vi "Standard Event Status Enable.vi"(0 "VISA resource name":refnum<visa-resource-name>, 5 "Standard Event Status Enable":T1, 11 "error in (no error)":errorcluster) -> (4 "VISA resource name out":refnum<visa-resource-name>, 15 "error out":errorcluster)   [LabVIEW 2014, in "Associated Power Technologies 8500 Series.lvlib"]
doc: "Enables the events for which the status is to be monitored in the instrument.\n\nThe Standard Event Register consists of the following 8 bits.\nBit 0: Operation Complete\nBit 1: not used\nBit 2: Query Error \nBit 3: Device Error\nBit 4: Message Available\nBit 5: Command Error \nBit 6: not used\nBit 7: Power On\n\nExample:\nIf the User gives 0|dec (whose binary equivalent is 00000000|bin) to this VI, no event status will be enabled.\n\nIf 255|dec (11111111|bin) is given, all the events (Operation Complete, User Defined, Query Error, Device Error, Message Available, Command Error,User Defined, Power On) will be enabled.\n\n<B>Default</B>: 32|dec=00100000|bin"
uses:
  <instrlib>/Associated Power Technologies 8500 Series/Associated Power Technologies 8500 Series.lvlib
panel:
  # "Bit 0: Operation Complete\nBit 1:  not used\nBit 2:  Query Error\t\nBit 3:  Device Error\nBit 4:\t\tMessage Available\nBit 5:  Command Error\t\nBit 6:  not used\nBit 7:  Power On"
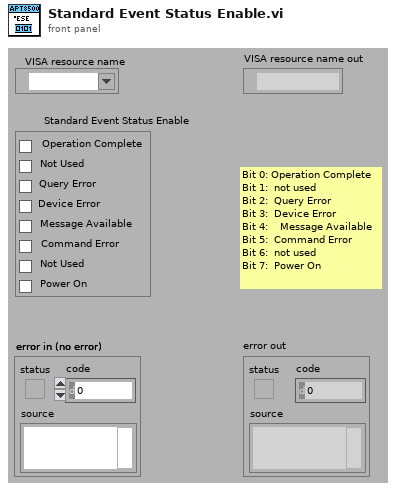
[diagram p1: front panel]
types:
  T1 = cluster{"Operation Complete":bool, "Not Used":bool, "Query Error":bool, "Device Error":bool, "Message Available":bool, "Command Error":bool, "Not Used":bool, "Power On":bool}
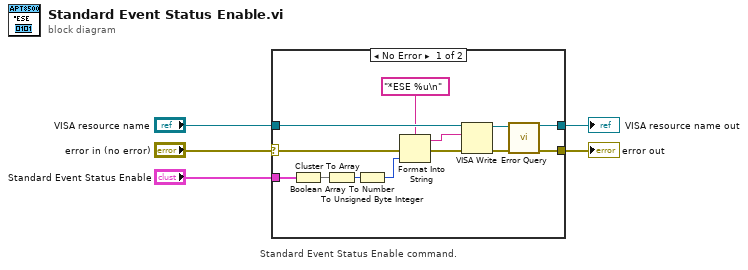
[diagram p0: block diagram]
diagram:
  # "Standard Event Status Enable command."
  n1 = case shown="No Error" "error in (no error)" {
    selector: "error in (no error)" -> [w12 w20]
    tunnel: "VISA resource name" -> [w18 w19]
    tunnel: [w16 w19] -> w5
    tunnel: [w14 w20] -> w4
    tunnel: "Standard Event Status Enable" -> [w8 _]
    frame No Error {
      n2 = Cluster To Array(cluster=w8) -> (array=w9:bool[])
      n3 = Boolean Array To Number(Boolean array=w9) -> (number=w7:u32)
      n4 = To Unsigned Byte Integer(number=w7) -> (unsigned 8bit integer=w6:u8)
      n5 = Format Into String(format string="*ESE %u\n" ("Command to Send"), error in=w12, w6) -> (resulting string=w13:string, error out=w11:errorcluster)  [unwired: 1 in]
      n6 = VISA Write(VISA resource name=w18, write buffer=w13, error in (no error)=w11) -> (VISA resource name out=w17:refnum<visa-resource-name>, error out=w15:errorcluster)  [unwired: 1 out]
      n7 = call <instrlib>:"Error Query.vi"("VISA resource name"=w17, "error in (no error)"=w15) -> ("VISA resource name out"=w16:refnum<visa-resource-name>, "error out"=w14:errorcluster)  [unwired: 10 in, 2 out]
    }
    frame Error {
    }
  }
  "error out" <- w4
  "VISA resource name out" <- w5
